vi "generate_and_save_phase_data.vi"() -> ()   [LabVIEW 2019]
uses:
  <vilib>/Utility/file.llb/Write Delimited Spreadsheet (DBL).vi
panel:
  in  "starting pixel":dbl=143.0 format="%#_13g"
  in  "Mask B Calibration Path":path=path "G:/My Drive/ansom/Data/THz 1/pulse shaping/SLM voltage calibration 28 June 2021/Mask_B_fine_calibration.txt"
  in  "Mask A Calibration Path":path=path "G:/My Drive/ansom/Data/THz 1/pulse shaping/Calibrations 22October21/Voltage Calibration Mask A.txt"
  in  "Mask B Data folder":path=path "G:/My Drive/ansom/Data/THz 1/pulse shaping/SLM voltage calibration 28 June 2021/Mask_B_phase_voltage"
  in  "Mask A Data folder":path=path "G:/My Drive/ansom/Data/THz 1/pulse shaping/Calibrations 22October21/Mask A conversion"
  # "Input: Calibration intensity plot file from initial program"
  # "Output: folders where voltage/phase curves for each pixel are saved"
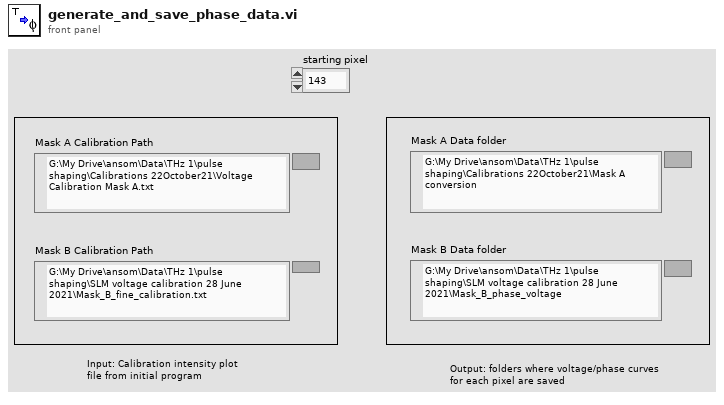
[diagram p1: front panel]
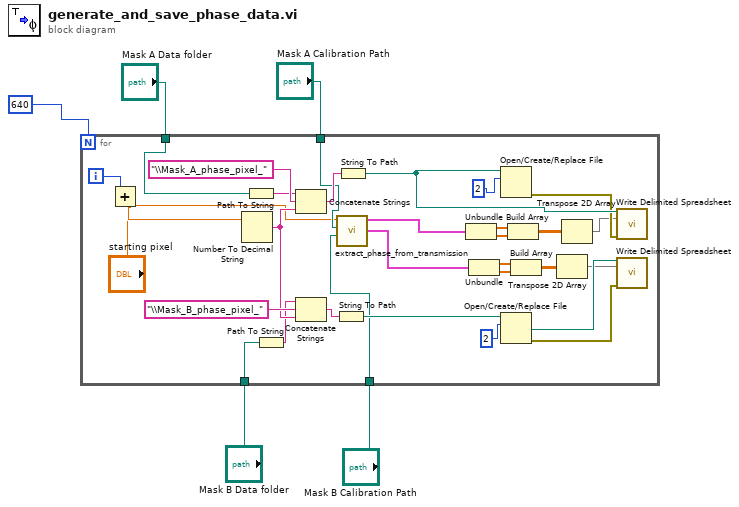
[diagram p0: block diagram]
diagram:
  n1 = for {
    N: 640 -> [_]
    tunnel: "Mask A Data folder" -> [w34]
    tunnel: "Mask B Data folder" -> [w22]
    tunnel: "Mask A Calibration Path" -> [w21]
    tunnel: "Mask B Calibration Path" -> [w20]
    i -> [w35]
    n2 = Add(x=w35, y="starting pixel") -> (x+y=w19:dbl)
    n3 = Number To Decimal String(number=w19) -> (decimal integer string=w29:string)  [unwired: 1 in]
    n4 = Path To String(path=w34) -> (string=w28:string)
    n5 = Path To String(path=w22) -> (string=w23:string)
    n6 = Concatenate Strings(w28, "\\Mask_A_phase_pixel_", w29) -> (w33:string)
    n7 = Concatenate Strings(w23, "\\Mask_B_phase_pixel_", w29) -> (w26:string)
    n8 = String To Path(string=w26) -> (path=w24:path)
    n9 = call "extract_phase_from_transmission.vi"("Mask B Calibration Path"=w20, "Mask A Calibration Path"=w21, "Pixel number"=w19) -> ("Mask B Phase"=w27:cluster{"Ramp Pattern":dbl[], "phase out":dbl[]}, "Mask A Phase"=w31:cluster{"Ramp Pattern":dbl[], "phase out":dbl[]})  [unwired: 7 in]
    n10 = String To Path(string=w33) -> (path=w25:path)
    n11 = Unbundle(w31) -> ("Ramp Pattern"=w16:dbl[], "phase out"=w15:dbl[])
    n12 = Unbundle(w27) -> ("Ramp Pattern"=w14:dbl[], "phase out"=w13:dbl[])
    n13 = Open/Create/Replace File(file path (use dialog)=w25, operation (0:open)=2) -> (error out=w12:errorcluster)  [unwired: 4 in, 2 out]
    n14 = Open/Create/Replace File(file path (use dialog)=w24, operation (0:open)=2) -> (error out=w11:errorcluster)  [unwired: 4 in, 2 out]
    n15 = Build Array(w16, w15) -> (w8:dbl[][])
    n16 = Build Array(w14, w13) -> (w9:dbl[][])
    n17 = Transpose 2D Array(2D array=w9) -> (transposed array=w6:dbl[][])
    n18 = Transpose 2D Array(2D array=w8) -> (transposed array=w7:dbl[][])
    n19 = call-poly <vilib>:"Write Delimited Spreadsheet.vi"("file path (dialog if empty)"=w25, "2D data"=w7, "error in (no error)"=w12) -> ()  [unwired: 11 in, 2 out]
    n20 = call-poly <vilib>:"Write Delimited Spreadsheet.vi"("file path (dialog if empty)"=w24, "2D data"=w6, "error in (no error)"=w11) -> ()  [unwired: 11 in, 2 out]
  }
